vi "Labview_Database_try_multi-channel one chart.vi"() -> ()   [LabVIEW 2012]
uses:
  <vilib>/addons/database/Connection.llb/DB Tools Open Connec (Path).vi
  <vilib>/addons/database/NI_Database_API.lvlib
panel:
  out "Plot":cluster{dbl[], dbl[]}[](graph)
  out "Temperature-Time Plot":cluster{dbl[], dbl[]}(graph)
  in  "Start time":timestamp
  in  "End time":timestamp
  out "Pressure-Time Plot":cluster{dbl[], dbl[]}(graph)
  out "data":string[][](table)
  out "error out":errorcluster
  in  "Table chosen":string
  in  "stop":bool
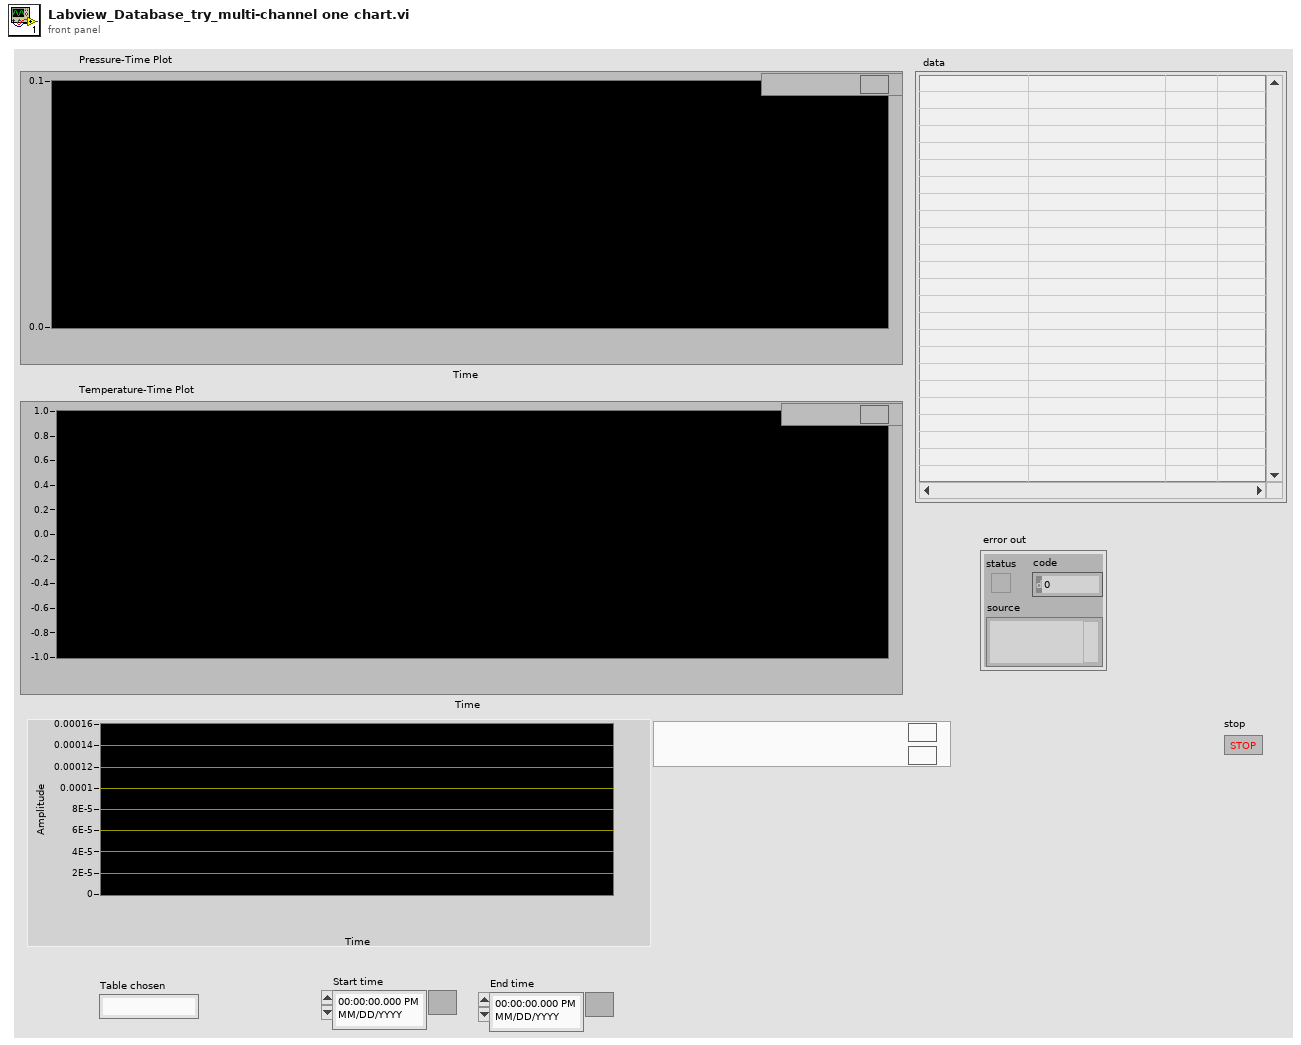
[diagram p1: front panel]
types:
  T1 = typedef "NI_Database_API.lvlib/Conn ObjectReference.ctl" = refnum<k1>
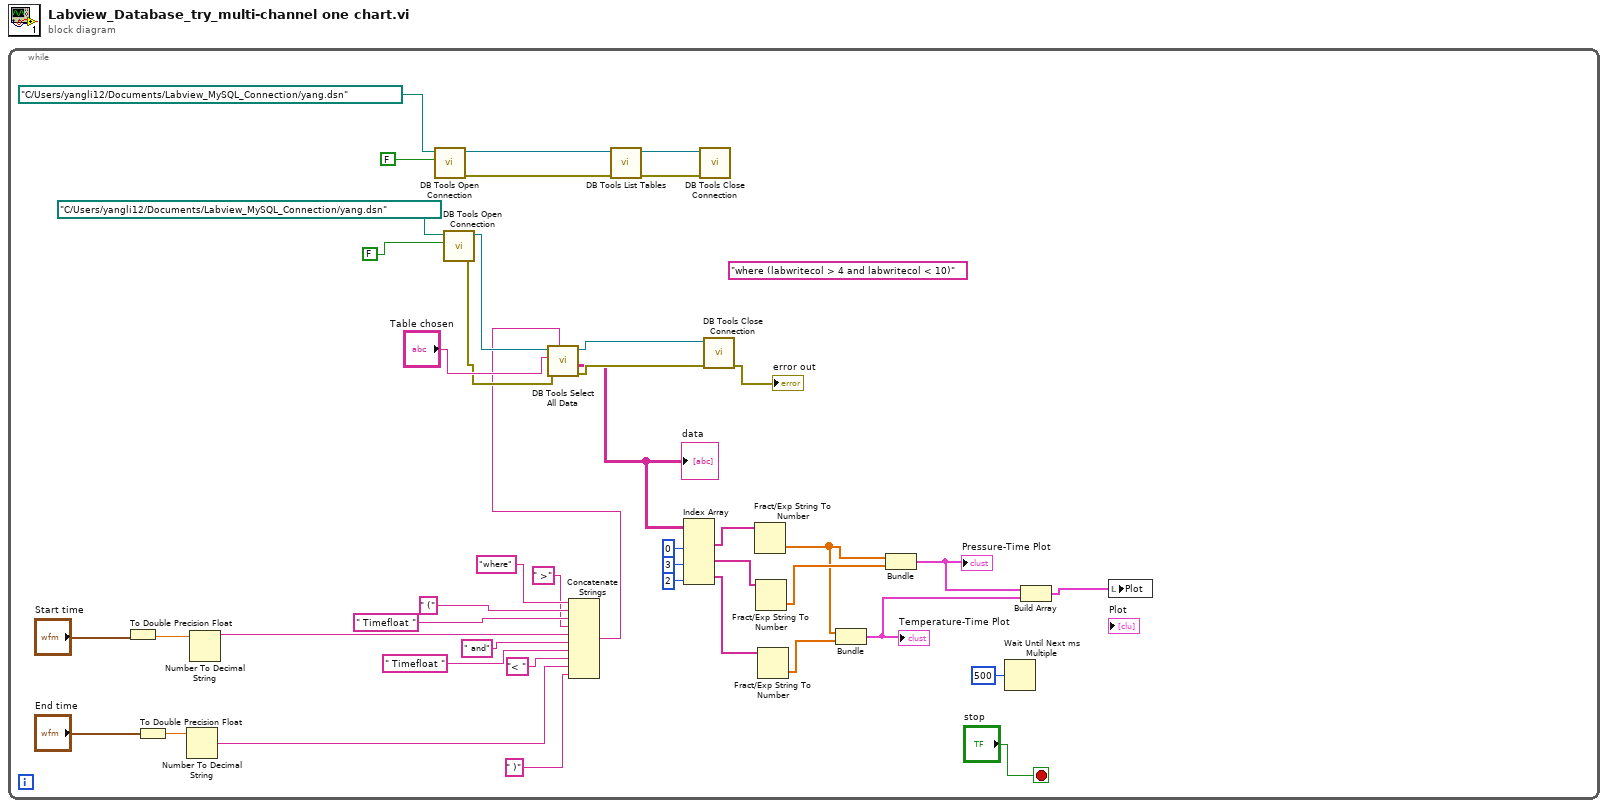
[diagram p0: block diagram]
diagram:
  n1 = while {
    stop <- "stop" stop-if-true
    (unwired) "where (labwritecol > 4 and labwritecol < 10)" ("condition")
    n2 = To Double Precision Float(number="Start time") -> (double precision float=w17:dbl)
    n3 = To Double Precision Float(number="End time") -> (double precision float=w12:dbl)
    n4 = Number To Decimal String(number=w12) -> (decimal integer string=w11:string)  [unwired: 1 out]
    n5 = Number To Decimal String(number=w17) -> (decimal integer string=w16:string)  [unwired: 1 out]
    n6 = call-poly <vilib>:"DB Tools Open Connection.vi"("prompt? (F)"=FALSE, "connection information"=path "C:/Users/yangli12/Documents/Labview_MySQL_Connection/yang.dsn") -> ("error out"=w37:errorcluster, "connection reference"=w38:T1)  [unwired: 6 in]
    n7 = call-poly <vilib>:"DB Tools Open Connection.vi"("prompt? (F)"=FALSE, "connection information"=path "C:/Users/yangli12/Documents/Labview_MySQL_Connection/yang.dsn") -> ("error out"=w31:errorcluster, "connection reference"=w33:T1)  [unwired: 6 in]
    n8 = Concatenate Strings("where", " (", " Timefloat " ("string"), " >" ("string"), w16, " and", " Timefloat ", "< " ("string"), w11, " )") -> (w9:string)
    n9 = call <vilib>:"DB Tools Select All Data.vi"("optional clause"=w9, "error in (no error)"=w31, "table"="Table chosen", "connection reference"=w33) -> ("error out"=w30:errorcluster, "data"=w28:string[][], "connection reference out"=w29:T1)  [unwired: 1 in, 1 out]
    "data" <- w28
    n10 = call <vilib>:"DB Tools List Tables.vi"("error in (no error)"=w37, "connection reference"=w38) -> ("error out"=w42:errorcluster, "connection reference out"=w43:T1)  [unwired: 3 in, 1 out]
    n11 = Index Array(array=w28, index (col) #1=0 ("disabled index (col)"), index (col) #2=3 ("index (col)"), index (col) #3=2 ("index (col)")) -> (element #1=w25:string[], element #2=w4:string[], element #3=w8:string[])  [unwired: 3 in]
    n12 = call <vilib>:"DB Tools Close Connection.vi"("error in (no error)"=w42, "connection reference"=w43) -> ()  [unwired: 5 in, 1 out]
    n13 = call <vilib>:"DB Tools Close Connection.vi"("error in (no error)"=w30, "connection reference"=w29) -> ("error out"=→"error out":errorcluster)  [unwired: 5 in]
    n14 = Fract/Exp String To Number(string=w25) -> (number=w7:dbl[])  [unwired: 4 out]
    n15 = Fract/Exp String To Number(string=w4) -> (number=w24:dbl[])  [unwired: 4 out]
    n16 = Fract/Exp String To Number(string=w8) -> (number=w6:dbl[])  [unwired: 4 out]
    n17 = Bundle "Bundle"(w7, w6) -> (w2:cluster{dbl[], dbl[]})  [unwired: 1 in]
    "Temperature-Time Plot" <- w2
    n18 = Bundle "Bundle"(w7, w24) -> (w3:cluster{dbl[], dbl[]})  [unwired: 1 in]
    "Pressure-Time Plot" <- w3
    n19 = Wait Until Next ms Multiple(millisecond multiple=u32 500) -> ()  [unwired: 1 out]
    n20 = Build Array(w3, w2) -> (w1:cluster{dbl[], dbl[]}[])
    n21 = local write "Plot"(w1) -> ()
  }
